vi "qFactorCalculator.vi"(9 "Step Size":dbl, 10 "Frequencies":dbl[](array[numeric]), 11 "Signal":dbl[](array[numeric])) -> (1 "Resonance Frequency":i32, 2 "FWHM":dbl, 3 "Q-Factor":dbl)   [LabVIEW 2016]
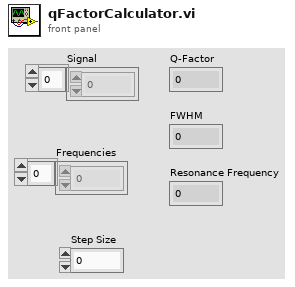
[diagram p1: front panel]
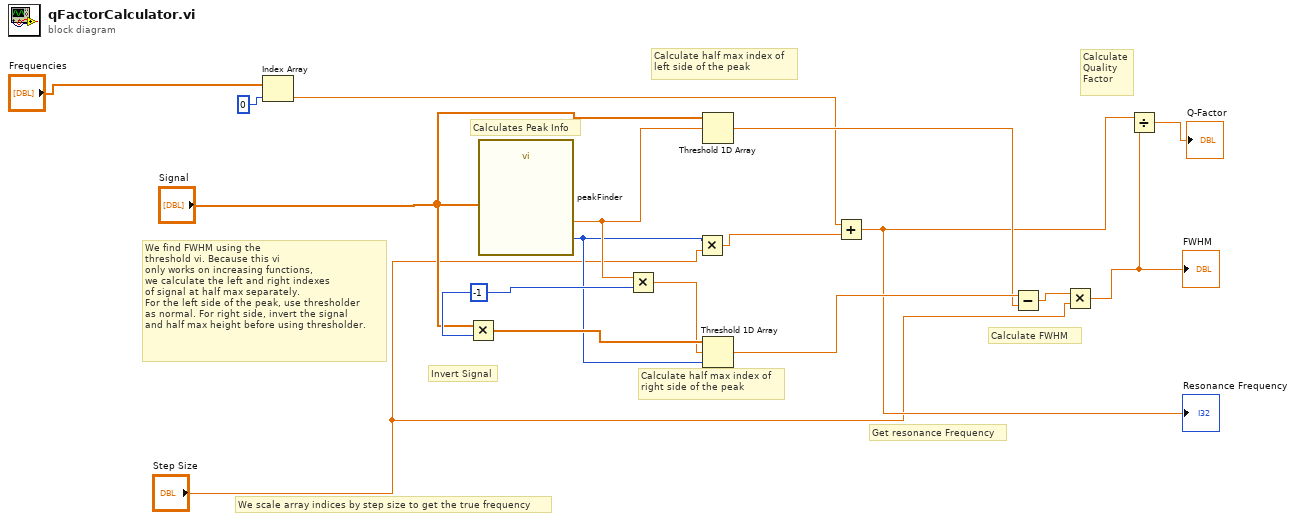
[diagram p0: block diagram]
diagram:
  w12 = -1
  # "We scale array indices by step size to get the true frequency"
  # "Get resonance Frequency"
  # "We find FWHM using the \nthreshold vi. Because this vi \nonly works on increasing functions,\nwe calculate the left and right indexes \nof signal at half max separately. \nFor the left side of the peak, use thresholder \nas normal. For right side, invert the signal\nand half max height before using thresholder."
  # "Calculate\nQuality \nFactor"
  # "Calculate FWHM"
  # "Calculate half max index of\nright side of the peak"
  # "Invert Signal"
  # "Calculate half max index of\nleft side of the peak"
  # "Calculates Peak Info"
  n1 = Index Array(array="Frequencies", index=0) -> (element=w4:dbl)
  n2 = Multiply(x="Signal", y=w12) -> (x*y=w14:dbl[])
  n3 = call "peakFinder.vi"("Input Signal"="Signal") -> ("Peak Index"=w6:i32, "Half Max Height"=w15:dbl)  [unwired: 9 in]
  n4 = Multiply(x=w15, y=w12) -> (x*y=w7:dbl)
  n5 = Multiply(x=w6, y="Step Size") -> (x*y=w5:dbl)
  n6 = Threshold 1D Array(2:w15, 3:"Signal") -> (0:w13:dbl)  [unwired: 1 in]
  n7 = Threshold 1D Array(1:w6, 2:w7, 3:w14) -> (0:w17:dbl)
  n8 = Add(x=w4, y=w5) -> (x+y=w8:dbl)
  "Resonance Frequency" <- w8
  n9 = Subtract(x=w17, y=w13) -> (x-y=w2:dbl)
  n10 = Multiply(x=w2, y="Step Size") -> (x*y=w1:dbl)
  "FWHM" <- w1
  n11 = Divide(x=w8, y=w1) -> (x/y=→"Q-Factor":dbl)
